vi "PromptToSave.vi"(6 "Working script":path, 7 "Config Cluster in":T1, 8 "error in":errorcluster, 9 "Script Saved?":bool, 10 "Script name":string) -> (0 "error out":errorcluster, 4 "Working Script out":path, 5 "Config Cluster out":T1)   [LabVIEW 2010]
uses:
  Config cluster.ctl
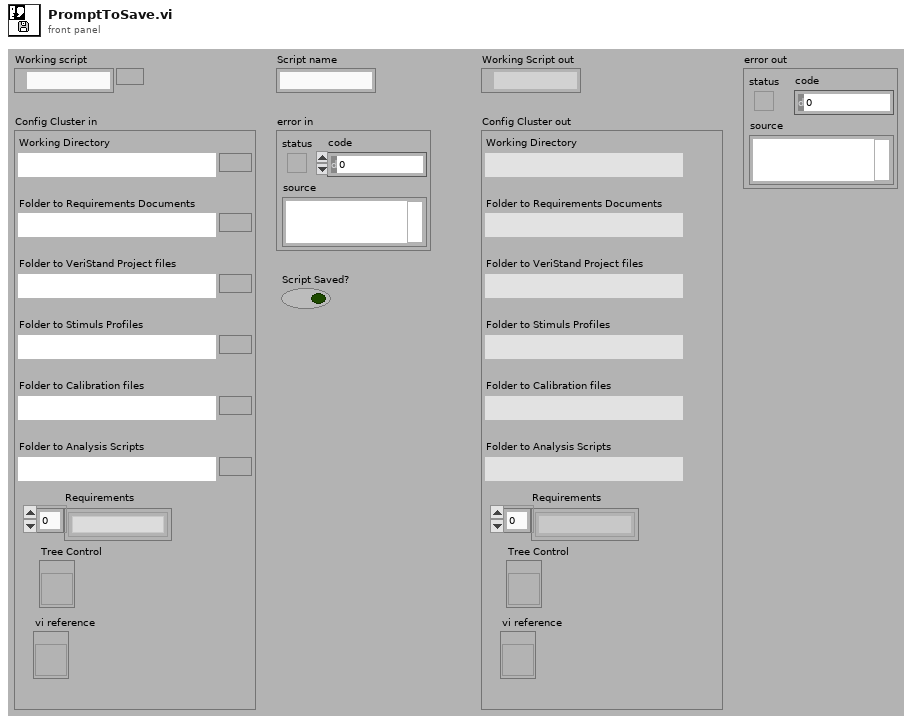
[diagram p1: front panel]
types:
  T1 = typedef "Config cluster.ctl" = cluster{"Working Directory":path, "Folder to Requirements Documents":path, "Folder to VeriStand Project files":path, "Folder to Stimuls Profiles":path, "Folder to Calibration files":path, "Folder to Analysis Scripts":path, "Requirements":string[], "Tree Control":refnum<vi>, "vi reference":refnum<vi>}
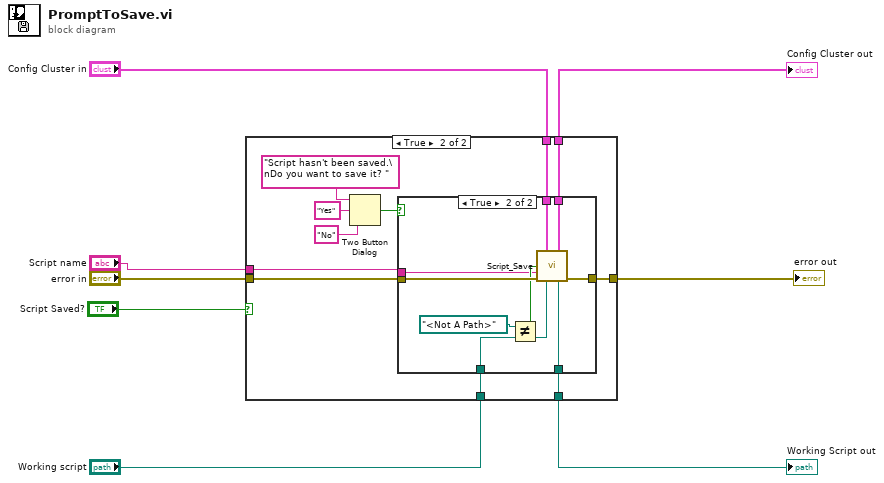
[diagram p0: block diagram]
diagram:
  n1 = case shown="True" "Script Saved?" {
    tunnel: "error in" -> [w11 w18]
    tunnel: [w11 w17] -> w3
    tunnel: "Working script" -> [w9 w16]
    tunnel: "Config Cluster in" -> [w10 w15]
    tunnel: [w10 w14] -> w5
    tunnel: [w9 w13] -> w7
    tunnel: "Script name" -> [_ w12]
    frame False {
    }
    frame True {
      n2 = Two Button Dialog(message="Script hasn't been saved.\nDo you want to save it? ", 1:"No" ("F button name (\"Cancel\")"), 2:"Yes" ("T button name (\"OK\")")) -> (T button?=w19:bool)
      n3 = case shown="True" w19 {
        tunnel: w18 -> [w25 w34]
        tunnel: [w25 w33] -> w17
        tunnel: w16 -> [w23 w28]
        tunnel: w15 -> [w24 w30]
        tunnel: [w24 w29] -> w14
        tunnel: [w23 w27] -> w13
        tunnel: w12 -> [_ w26]
        frame False {
        }
        frame True {
          n4 = Not Equal?(x=path "<Not A Path>" ("selected path"), y=w28) -> (x != y?=w31:bool)
          n5 = call "Script_Save.vi"("Config Cluster in"=w30, "Save/SaveAs(Save= True)"=w31, "Script name"=w26, "error in"=w34, "Working Script"=w28) -> ("Config Cluster out"=w29:T1, "Working Script out"=w27:path, "error out"=w33:errorcluster)  [unwired: 5 in, 3 out]
        }
      }
    }
  }
  "Working Script out" <- w7
  "Config Cluster out" <- w5
  "error out" <- w3
